vi "Autofeed.vi"(4 "duration":dbl format="%.4f", 5 "Auto-feed":cluster{"Fix":dbl, "Rnd":dbl}={"Fix"=0.18, "Rnd"=0.0} {"Rnd" format="%.4f"; "Fix" format="%_4g"}, 6 "DO Task":refnum<k21>="BlueSimple_DO") -> ()   [LabVIEW 2010]
panel:
  # "+"
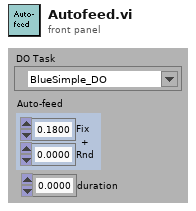
[diagram p1: front panel]
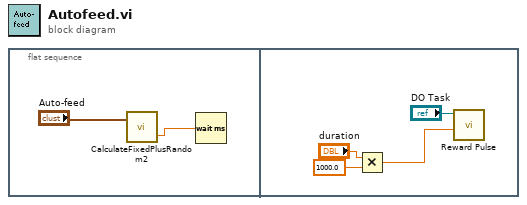
[diagram p0: block diagram]
diagram:
  n1 = flat-sequence {
    frame #0 {
      n2 = call "CalculateFixedPlusRandom2.vi"("Component times"="Auto-feed") -> ("time in ms"=w1:dbl)  [unwired: 1 in, 1 out]
      n3 = Wait (ms)(milliseconds to wait=w1) -> ()  [unwired: 1 out]
    }
    frame #1 {
      n4 = Multiply(x="duration", y=1000.0) -> (x*y=w4:dbl)
      n5 = call "Reward Pulse.vi"("Pulse duration (ms)"=w4, "DO Task"="DO Task") -> ()  [unwired: 8 in]
    }
  }
